vi "Config filepath ---constant.vi"() -> (3 "config file path":path)   [LabVIEW 2020]
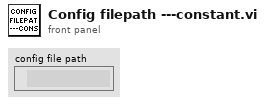
[diagram p1: front panel]
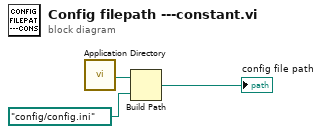
[diagram p0: block diagram]
diagram:
  n1 = call <vilib>:"Application Directory.vi"() -> ("Application Directory"=w2:path)
  n2 = Build Path(base path=w2, name or relative path=path "config/config.ini") -> (appended path=→"config file path":path)
